vi "InShotTimeWindow.vi"(1 "Charge Step":T1(ring), 2 "Running  \nShot \nSequence":bool, 3 "Turn IG back on after shot (s)":dbl format="%#_13g", 4 "Time Since Shot (s)":dbl format="%#_13g") -> (0 "In Shot Time Window":bool)   [LabVIEW 2016]
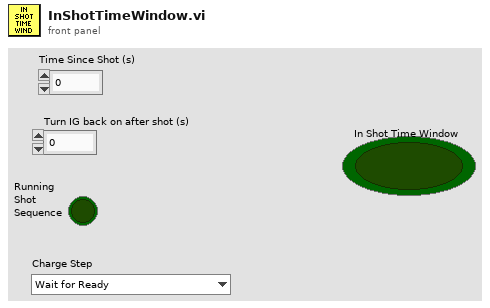
[diagram p1: front panel]
types:
  T1 = enum16{"Wait for Ready", "Prep for Charge", "Open Dump Relays", "Close Connect Relays", "Wait PS Delays", "Wait End of Charge", "Turn Off HV", "Open Connect Relays", "Charge Done"}
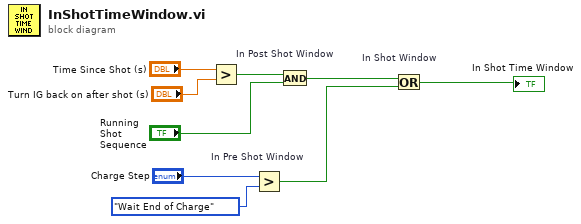
[diagram p0: block diagram]
diagram:
  n1 = Greater?(x="Time Since Shot (s)", y="Turn IG back on after shot (s)") -> (0:w5:bool)
  n2 = Greater? "In Pre Shot Window"(x="Charge Step", y=T1."Wait End of Charge") -> (0:w2:bool)
  n3 = And "In Post Shot Window"(x=w5, y="Running  \nShot \nSequence") -> (x .and. y?=w3:bool)
  n4 = Or "In Shot Window"(x=w3, y=w2) -> (x .or. y?=→"In Shot Time Window":bool)
